vi "_refMgrTerms.vi"(1 "type":T1, 2 "Single?":bool, 3 "Type":variant) -> (0 "Array":T2[](array[typedef]))   [LabVIEW 2014, in "RefManager(dev).lvlib"]
uses:
  RefManager(dev).lvlib
  <vilib>/XNodeSupport/XNodeTerm4.ctl
  <vilib>/XNodeSupport/XNodeString.ctl
  <vilib>/XNodeSupport/XNodeVariant.ctl
  <vilib>/XNodeSupport/XNodeRect32.ctl
  <vilib>/XNodeSupport/XNodeInt.ctl
  <vilib>/XNodeSupport/XNodeBool.ctl
  <vilib>/XNodeSupport/XNodeTermDirection.ctl
  _refMgrFunc.ctl
  <vilib>/XNodeSupport/NI_XNodeSupport.lvlib
  <userlib>/_NEVSTOP/TagDB/Core/TagDB.lvlib
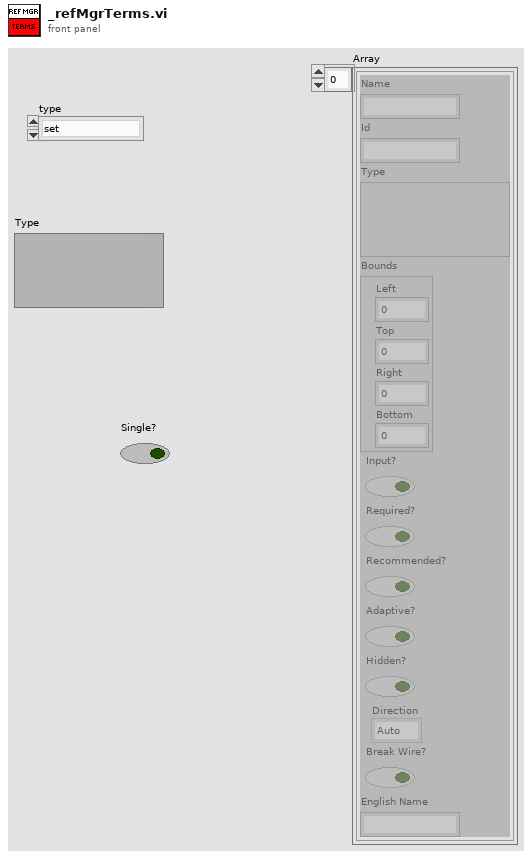
[diagram p1: front panel]
types:
  T1 = typedef "RefManager(dev).lvlib/_refMgrFunc.ctl" = enum16{"set", "get", "reset", "remove"}
  T2 = typedef "NI_XNodeSupport.lvlib/XNodeTerm4.ctl" = cluster{"Name":T3, "Id":T3, "Type":T4, "Bounds":T5, "Input?":T7, "Required?":T7, "Recommended?":T7, "Adaptive?":T7, "Hidden?":T7, "Direction":T8, "Break Wire?":T7, "English Name":T3}
  T3 = typedef "NI_XNodeSupport.lvlib/XNodeString.ctl" = string
  T4 = typedef "NI_XNodeSupport.lvlib/XNodeVariant.ctl" = variant
  T5 = typedef "NI_XNodeSupport.lvlib/XNodeRect32.ctl" = cluster{"Left":T6, "Top":T6, "Right":T6, "Bottom":T6}
  T6 = typedef "NI_XNodeSupport.lvlib/XNodeInt.ctl" = i32
  T7 = typedef "NI_XNodeSupport.lvlib/XNodeBool.ctl" = bool
  T8 = typedef "NI_XNodeSupport.lvlib/XNodeTermDirection.ctl" = enum32{"Auto", "Up", "Down", "Left", "Right", "Center"}
  T9 = typedef "TagDB.lvlib/tagDB_Def.ctl" = refnum<k1>
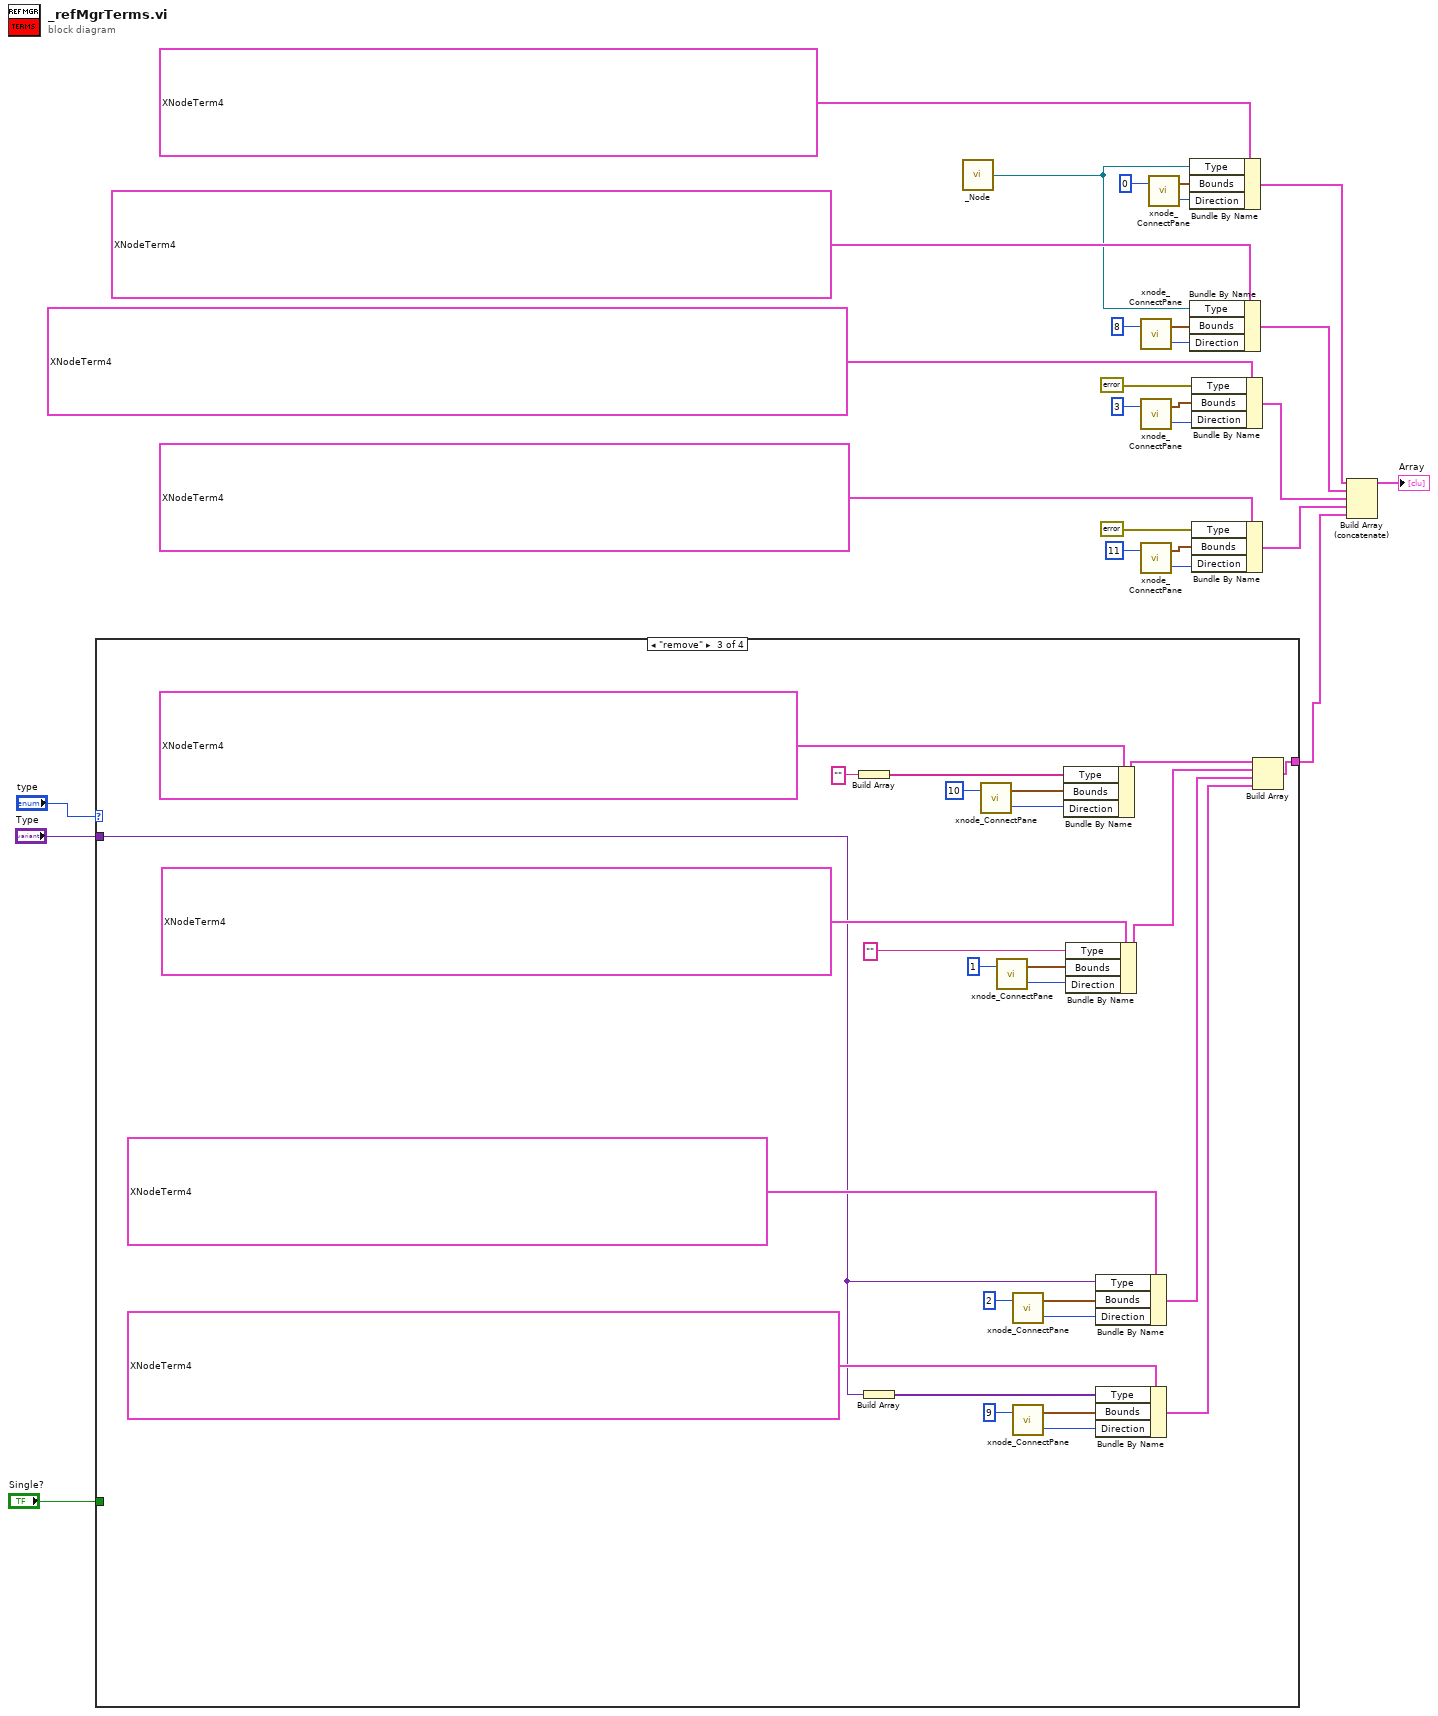
[diagram p0: block diagram]
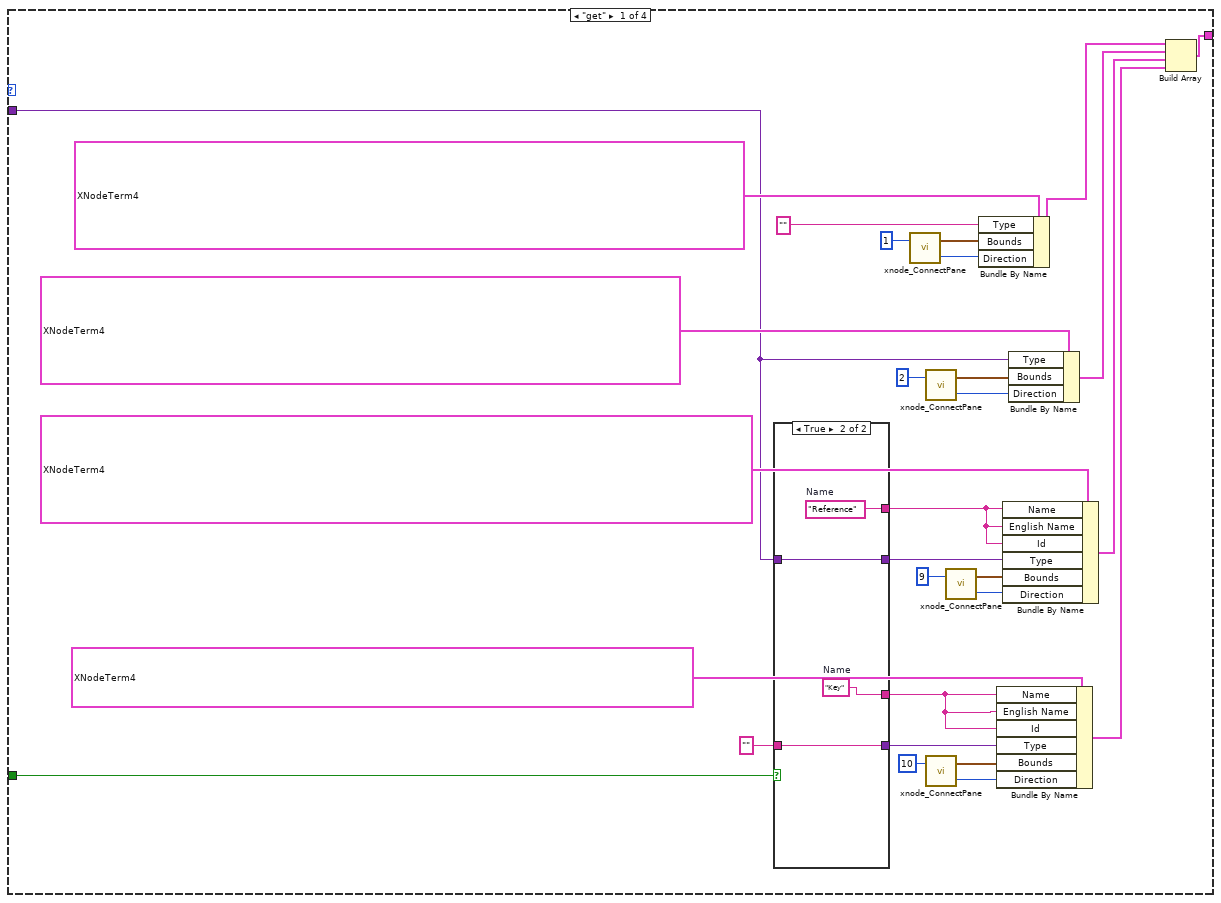
[diagram p2: hidden frame]
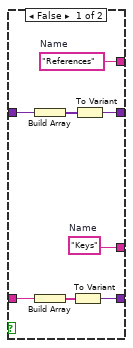
[diagram p3: hidden frame]
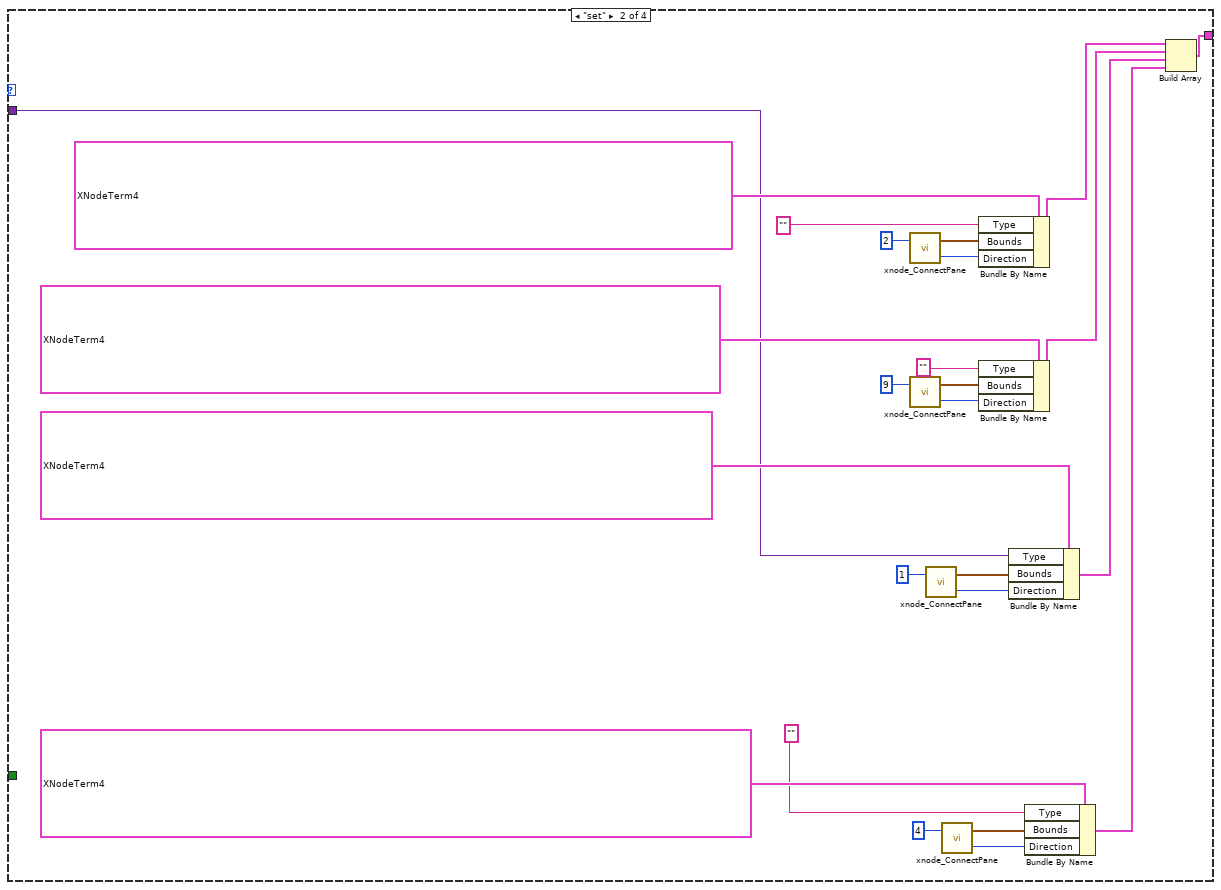
[diagram p4: hidden frame]
diagram:
  n1 = case shown="\"remove\"" "type" {
    tunnel: [w57 w94 w120 _] -> w17
    tunnel: "Type" -> [w49 w86 w112 _]
    tunnel: "Single?" -> [w32 _ _ _]
    frame "get" {
      n2 = case shown="True" w32 {
        tunnel: w49 -> [w65 w68]
        tunnel: [w60 w68] -> w36
        tunnel: [w61 w69] -> w35
        tunnel: "" -> [w63 w69]
        tunnel: [w59 w66] -> w30
        tunnel: [w58 w67] -> w29
        frame False {
          w58 = T3 "Keys"  # Name
          w59 = T3 "References"  # Name
          n3 = Build Array(w65) -> (w64:variant[])
          n4 = Build Array(w63) -> (w62:string[])
          n5 = To Variant(anything=w62) -> (Variant=w61:variant)
          n6 = To Variant(anything=w64) -> (Variant=w60:variant)
        }
        frame True {
          w66 = T3 "Reference"  # Name
          w67 = T3 "Key"  # Name
        }
      }
      n7 = call <userlib>:"xnode_ConnectPane.vi"("index"=1) -> ("Direction"=w47:T8, "Bounds"=w46:T5)  [unwired: 1 in]
      n8 = call <userlib>:"xnode_ConnectPane.vi"("index"=2) -> ("Direction"=w41:T8, "Bounds"=w40:T5)  [unwired: 1 in]
      n9 = call <userlib>:"xnode_ConnectPane.vi"("index"=10) -> ("Direction"=w38:T8, "Bounds"=w37:T5)  [unwired: 1 in]
      n10 = call <userlib>:"xnode_ConnectPane.vi"("index"=9) -> ("Direction"=w44:T8, "Bounds"=w43:T5)  [unwired: 1 in]
      n11 = Bundle By Name(cluster=T2 {"Name"="RegExp", "Id"="RegExp", "Type"=variant, "Bounds"={"Left"=0, "Top"=8, "Right"=0, "Bottom"=16}, "Input?"=TRUE, "Required?"=TRUE, "Recommended?"=FALSE, "Adaptive?"=FALSE, "Hidden?"=FALSE, "Direction"=enum."Left", "Break Wire?"=FALSE, "English Name"="RegExp"} ("Term 4"), "Type"="", "Bounds"=w46, "Direction"=w47) -> (w55:T2)
      n12 = Bundle By Name(cluster=T2 {"Name"="Keys", "Id"="Keys", "Type"=variant, "Bounds"={"Left"=32, "Top"=16, "Right"=32, "Bottom"=24}, "Input?"=FALSE, "Required?"=FALSE, "Recommended?"=TRUE, "Adaptive?"=TRUE, "Hidden?"=FALSE, "Direction"=enum."Right", "Break Wire?"=FALSE, "English Name"="Keys"} ("Term 4"), "Name"=w29, "English Name"=w29, "Id"=w29, "Type"=w35, "Bounds"=w37, "Direction"=w38) -> (w50:T2)
      n13 = Bundle By Name(cluster=T2 {"Name"="References", "Id"="References", "Type"=variant, "Bounds"={"Left"=32, "Top"=8, "Right"=32, "Bottom"=16}, "Input?"=FALSE, "Required?"=FALSE, "Recommended?"=TRUE, "Adaptive?"=TRUE, "Hidden?"=FALSE, "Direction"=enum."Right", "Break Wire?"=FALSE, "English Name"="References"} ("Term 4"), "Name"=w30, "English Name"=w30, "Id"=w30, "Type"=w36, "Bounds"=w43, "Direction"=w44) -> (w33:T2)
      n14 = Bundle By Name(cluster=T2 {"Name"="Type", "Id"="Type", "Type"=variant, "Bounds"={"Left"=4, "Top"=0, "Right"=12, "Bottom"=0}, "Input?"=TRUE, "Required?"=TRUE, "Recommended?"=FALSE, "Adaptive?"=TRUE, "Hidden?"=FALSE, "Direction"=enum."Up", "Break Wire?"=FALSE, "English Name"="Type"} ("Term 4"), "Type"=w49, "Bounds"=w40, "Direction"=w41) -> (w34:T2)
      n15 = Build Array(w55, w34, w33, w50) -> (w57:T2[])
    }
    frame "set" {
      n16 = call <userlib>:"xnode_ConnectPane.vi"("index"=2) -> ("Direction"=w81:T8, "Bounds"=w80:T5)  [unwired: 1 in]
      n17 = call <userlib>:"xnode_ConnectPane.vi"("index"=9) -> ("Direction"=w78:T8, "Bounds"=w77:T5)  [unwired: 1 in]
      n18 = call <userlib>:"xnode_ConnectPane.vi"("index"=1) -> ("Direction"=w75:T8, "Bounds"=w74:T5)  [unwired: 1 in]
      n19 = call <userlib>:"xnode_ConnectPane.vi"("index"=4) -> ("Direction"=w72:T8, "Bounds"=w71:T5)  [unwired: 1 in]
      n20 = Bundle By Name(cluster=T2 {"Name"="Name", "Id"="Name", "Type"=variant, "Bounds"={"Left"=0, "Top"=8, "Right"=0, "Bottom"=16}, "Input?"=TRUE, "Required?"=FALSE, "Recommended?"=TRUE, "Adaptive?"=FALSE, "Hidden?"=FALSE, "Direction"=enum."Left", "Break Wire?"=FALSE, "English Name"="Name"} ("Term 4"), "Type"="", "Bounds"=w80, "Direction"=w81) -> (w92:T2)
      n21 = Bundle By Name(cluster=T2 {"Name"="Ref-Key", "Id"="Ref-Key", "Type"=variant, "Bounds"={"Left"=32, "Top"=8, "Right"=32, "Bottom"=16}, "Input?"=FALSE, "Required?"=FALSE, "Recommended?"=TRUE, "Adaptive?"=FALSE, "Hidden?"=FALSE, "Direction"=enum."Right", "Break Wire?"=FALSE, "English Name"="Ref-Key"} ("Term 4"), "Type"="", "Bounds"=w77, "Direction"=w78) -> (w89:T2)
      n22 = Bundle By Name(cluster=T2 {"Name"="Refnum", "Id"="Refnum", "Type"=variant, "Bounds"={"Left"=4, "Top"=0, "Right"=12, "Bottom"=0}, "Input?"=TRUE, "Required?"=TRUE, "Recommended?"=FALSE, "Adaptive?"=TRUE, "Hidden?"=FALSE, "Direction"=enum."Up", "Break Wire?"=FALSE, "English Name"="Refnum"} ("Term 4"), "Type"=w86, "Bounds"=w74, "Direction"=w75) -> (w87:T2)
      n23 = Bundle By Name(cluster=T2 {"Name"="parentURL", "Id"="parentURL", "Type"=variant, "Bounds"={"Left"=4, "Top"=32, "Right"=12, "Bottom"=32}, "Input?"=TRUE, "Required?"=FALSE, "Recommended?"=TRUE, "Adaptive?"=FALSE, "Hidden?"=FALSE, "Direction"=enum."Down", "Break Wire?"=FALSE, "English Name"="parentURL"} ("Term 4"), "Type"="", "Bounds"=w71, "Direction"=w72) -> (w84:T2)
      n24 = Build Array(w92, w89, w87, w84) -> (w94:T2[])
    }
    frame "remove" {
      n25 = Build Array("") -> (w107:string[])
      n26 = Build Array(w112) -> (w111:variant[])
      n27 = call <userlib>:"xnode_ConnectPane.vi"("index"=10) -> ("Direction"=w105:T8, "Bounds"=w104:T5)  [unwired: 1 in]
      n28 = call <userlib>:"xnode_ConnectPane.vi"("index"=1) -> ("Direction"=w102:T8, "Bounds"=w101:T5)  [unwired: 1 in]
      n29 = call <userlib>:"xnode_ConnectPane.vi"("index"=2) -> ("Direction"=w99:T8, "Bounds"=w98:T5)  [unwired: 1 in]
      n30 = call <userlib>:"xnode_ConnectPane.vi"("index"=9) -> ("Direction"=w96:T8, "Bounds"=w95:T5)  [unwired: 1 in]
      n31 = Bundle By Name(cluster=T2 {"Name"="Keys", "Id"="Keys", "Type"=variant, "Bounds"={"Left"=20, "Top"=0, "Right"=28, "Bottom"=0}, "Input?"=FALSE, "Required?"=FALSE, "Recommended?"=TRUE, "Adaptive?"=FALSE, "Hidden?"=FALSE, "Direction"=enum."Up", "Break Wire?"=FALSE, "English Name"="Keys"} ("Term 4"), "Type"=w107, "Bounds"=w104, "Direction"=w105) -> (w108:T2)
      n32 = Bundle By Name(cluster=T2 {"Name"="RegExp", "Id"="RegExp", "Type"=variant, "Bounds"={"Left"=0, "Top"=8, "Right"=0, "Bottom"=16}, "Input?"=TRUE, "Required?"=TRUE, "Recommended?"=FALSE, "Adaptive?"=FALSE, "Hidden?"=FALSE, "Direction"=enum."Left", "Break Wire?"=FALSE, "English Name"="RegExp"} ("Term 4"), "Type"="", "Bounds"=w101, "Direction"=w102) -> (w118:T2)
      n33 = Bundle By Name(cluster=T2 {"Name"="Type", "Id"="Type", "Type"=variant, "Bounds"={"Left"=4, "Top"=0, "Right"=12, "Bottom"=0}, "Input?"=TRUE, "Required?"=TRUE, "Recommended?"=FALSE, "Adaptive?"=TRUE, "Hidden?"=FALSE, "Direction"=enum."Up", "Break Wire?"=FALSE, "English Name"="Type"} ("Term 4"), "Type"=w112, "Bounds"=w98, "Direction"=w99) -> (w115:T2)
      n34 = Bundle By Name(cluster=T2 {"Name"="References", "Id"="References", "Type"=variant, "Bounds"={"Left"=32, "Top"=16, "Right"=32, "Bottom"=24}, "Input?"=FALSE, "Required?"=FALSE, "Recommended?"=TRUE, "Adaptive?"=TRUE, "Hidden?"=FALSE, "Direction"=enum."Right", "Break Wire?"=FALSE, "English Name"="References"} ("Term 4"), "Type"=w111, "Bounds"=w95, "Direction"=w96) -> (w113:T2)
      n35 = Build Array(w108, w118, w115, w113) -> (w120:T2[])
    }
    frame "reset" {
    }
  }
  n36 = call <userlib>:"_Node.vi"() -> ("TagDB Node"=w1:T9)  [unwired: 1 in]
  n37 = call <userlib>:"xnode_ConnectPane.vi"("index"=8) -> ("Direction"=w10:T8, "Bounds"=w9:T5)  [unwired: 1 in]
  n38 = call <userlib>:"xnode_ConnectPane.vi"("index"=3) -> ("Direction"=w7:T8, "Bounds"=w6:T5)  [unwired: 1 in]
  n39 = call <userlib>:"xnode_ConnectPane.vi"("index"=11) -> ("Direction"=w4:T8, "Bounds"=w3:T5)  [unwired: 1 in]
  n40 = call <userlib>:"xnode_ConnectPane.vi"("index"=0) -> ("Direction"=w13:T8, "Bounds"=w14:T5)  [unwired: 1 in]
  n41 = Bundle By Name(cluster=T2 {"Name"="DB Ref", "Id"="DB Ref", "Type"=variant, "Bounds"={"Left"=0, "Top"=0, "Right"=8, "Bottom"=8}, "Input?"=TRUE, "Required?"=TRUE, "Recommended?"=FALSE, "Adaptive?"=FALSE, "Hidden?"=FALSE, "Direction"=enum."Left", "Break Wire?"=FALSE, "English Name"="DB Ref"} ("Term 4"), "Type"=w1, "Bounds"=w14, "Direction"=w13) -> (w19:T2)
  n42 = Bundle By Name(cluster=T2 {"Name"="DB Ref(dup)", "Id"="DB Ref(dup)", "Type"=variant, "Bounds"={"Left"=0, "Top"=0, "Right"=32, "Bottom"=8}, "Input?"=FALSE, "Required?"=FALSE, "Recommended?"=TRUE, "Adaptive?"=FALSE, "Hidden?"=FALSE, "Direction"=enum."Right", "Break Wire?"=FALSE, "English Name"="DB Ref(dup)"} ("Term 4"), "Type"=w1, "Bounds"=w9, "Direction"=w10) -> (w28:T2)
  n43 = Bundle By Name(cluster=T2 {"Name"="error in (no error)", "Id"="error in (no error)", "Type"=variant, "Bounds"={"Left"=0, "Top"=24, "Right"=0, "Bottom"=32}, "Input?"=TRUE, "Required?"=FALSE, "Recommended?"=TRUE, "Adaptive?"=FALSE, "Hidden?"=FALSE, "Direction"=enum."Left", "Break Wire?"=FALSE, "English Name"="error in (no error)"} ("Term 4"), "Type"=errorcluster {"status"=FALSE, "code"=0, "source"=""} ("error constant"), "Bounds"=w6, "Direction"=w7) -> (w22:T2)
  n44 = Bundle By Name(cluster=T2 {"Name"="error out", "Id"="error out", "Type"=variant, "Bounds"={"Left"=32, "Top"=24, "Right"=32, "Bottom"=32}, "Input?"=FALSE, "Required?"=FALSE, "Recommended?"=TRUE, "Adaptive?"=FALSE, "Hidden?"=FALSE, "Direction"=enum."Right", "Break Wire?"=FALSE, "English Name"="error out"} ("Term 4"), "Type"=errorcluster {"status"=FALSE, "code"=0, "source"=""} ("error constant"), "Bounds"=w3, "Direction"=w4) -> (w26:T2)
  n45 = Build Array (concatenate)(w19, w28, w22, w26, w17) -> (→"Array":T2[])
